vi "CONFOCAL MICROSCOPE.vi"() -> ()   [LabVIEW 2025]
uses:
  <vilib>/Analysis/1siggen.llb/Ramp Pattern by Samples.vi
  <vilib>/DAQmx/write.llb/DAQmx Write (Analog 1D Wfm NChan NSamp).vi
  <vilib>/DAQmx/read.llb/DAQmx Read (Counter 1D U32 1Chan NSamp).vi
  <vilib>/DAQmx/create/channels.llb/DAQmx Create Channel (AO-Voltage-Basic).vi
  <vilib>/DAQmx/configure/timing.llb/DAQmx Timing (Sample Clock).vi
  <vilib>/DAQmx/configure/events/hardwareSignals.llb/DAQmx Export Signal (Most Signals).vi
  <vilib>/DAQmx/miscellaneous.llb/DAQmx Fill In Error Info.vi
  <vilib>/DAQmx/create/channels.llb/DAQmx Create Channel (CI-Count Edges).vi
  <vilib>/Analysis/NI_AALBase.lvlib
panel:
  out "Sanning \nhas\nstarted":bool
  in  "Info Filling":bool
  in  "Length of the material":dbl
  in  "Objective magnification":dbl
  in  "Imaging focal length":dbl
  in  "Scaling factor":dbl
  in  "Pixel per line (X and Y)":dbl
  out "Resolution limit exceeded":bool
  out "transposed array":dbl[][](array[numeric])
  out "Intensity Graph":dbl[][](graph)
  out "Min Voltage (V)":dbl
  out "Max Voltage (V)":dbl
  in  "Dwell time (s)":dbl
  in  "Galvo mirror path":string
  in  "Sample mode":i32(ring)=10178 items=["Finite Samples"=10178, "Continuous Samples"=10123, "Hardware Timed Single Point"=12522]
  out "appended array":dbl[][](array[numeric])
  in  "Counter path":string
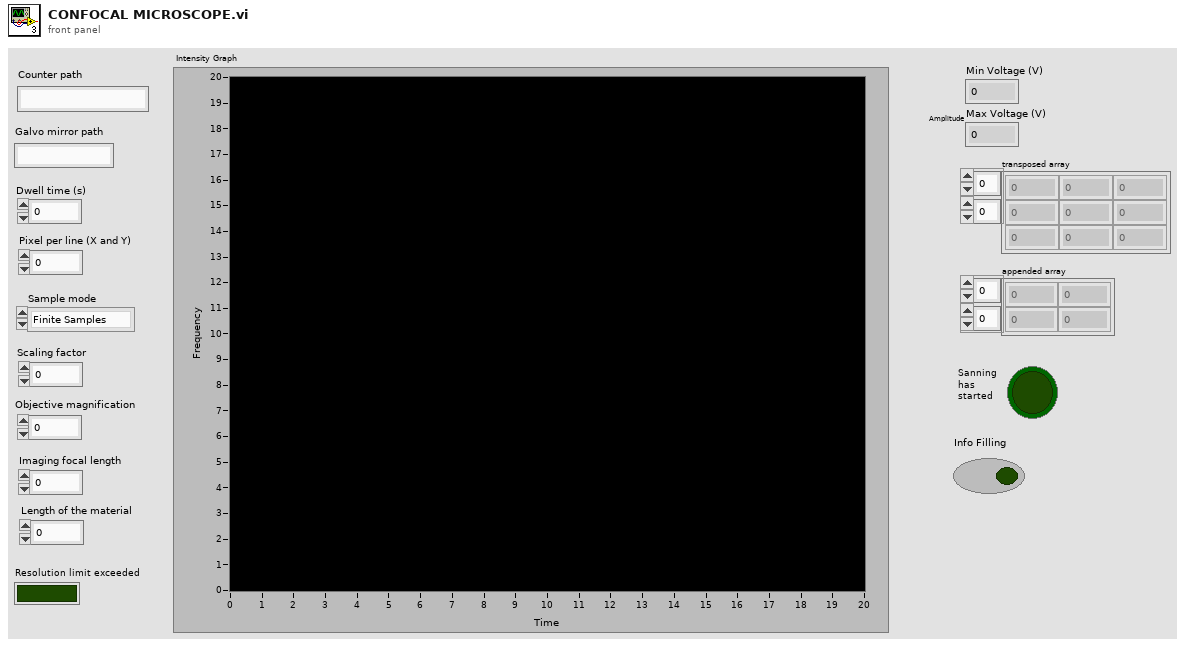
[diagram p1: front panel]
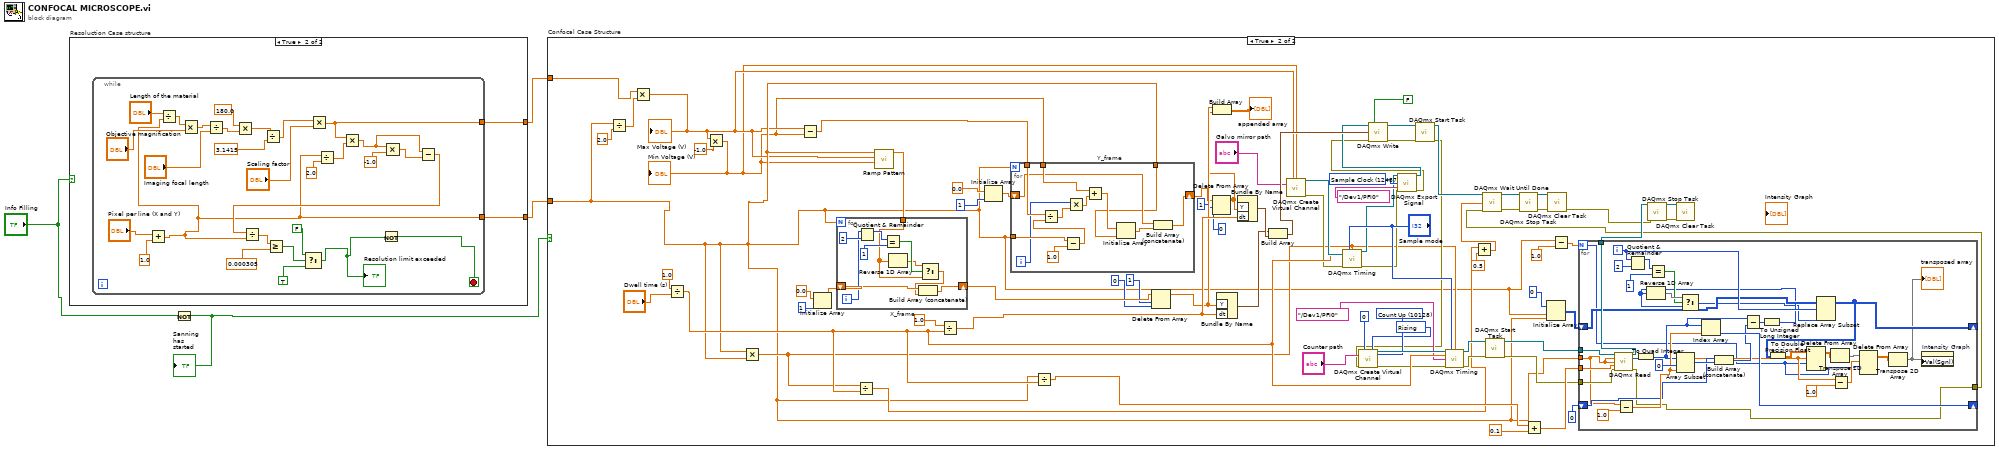
[diagram p0: block diagram]
diagram:
  n1 = case "Resoluction Case structure" shown="True" "Info Filling" {
    tunnel: [_ w5] -> w4
    tunnel: [_ w6] -> w3
    frame False {
    }
    frame True {
      n2 = while {
        tunnel: [w18] -> w6
        tunnel: [w7] -> w5
        stop <- w10 stop-if-true
        n3 = Add(x="Pixel per line (X and Y)", y=1.0) -> (x+y=w7:dbl)
        n4 = Divide(x="Length of the material", y=w7) -> (x/y=w33:dbl)
        n5 = Multiply(x=w33, y="Objective magnification") -> (x*y=w31:dbl)
        n6 = Divide(x=w31, y="Imaging focal length") -> (x/y=w28:dbl)
        n7 = Multiply(x=180.0, y=w28) -> (x*y=w27:dbl)
        n8 = Divide(x=w27, y=3.1415) -> (x/y=w25:dbl)
        n9 = Multiply(x=w25, y="Scaling factor") -> (x*y=w18:dbl)
        n10 = Divide(x=w7, y=2.0) -> (x/y=w17:dbl)
        n11 = Multiply(x=w18, y=w17) -> (x*y=w13:dbl)
        n12 = Multiply(x=w13, y=-1.0) -> (x*y=w14:dbl)
        n13 = Subtract(x=w13, y=w14) -> (x-y=w12:dbl)
        n14 = Divide(x=w12, y=w7) -> (x/y=w23:dbl)
        n15 = Greater Or Equal?(x=w23, y=0.000305) -> (x >= y?=w21:bool)
        n16 = Select(t=FALSE, s=w21, f=TRUE) -> (s? t:f=w11:bool)
        "Resolution limit exceeded" <- w11
        n17 = Not(x=w11) -> (.not. x?=w10:bool)
      }
    }
  }
  n18 = Not(x="Info Filling") -> (.not. x?=w1:bool)
  "Sanning \nhas\nstarted" <- w1
  n19 = case "Confocal Case Structure" shown="True" w1 {
    tunnel: w4 -> [_ w38]
    tunnel: w3 -> [_ w39]
    frame False {
    }
    frame True {
      w79 = 12487 items=["AI Convert Clock"=12484, "10MHz Reference Clock"=12536, "20MHz Timebase Clock"=12486, "Sample Clock"=12487, "Advance Trigger"=12488, "Reference Trigger"=12490, "Start Trigger"=12491, "Advance Complete Event"=12492, "AI Hold Complete Event"=12493, "Counter Output Event"=12494, "Change Detection Event"=12511, "Watchdog Timer Expired Event"=12512] ("signal")
      w84 = 10280 items=["Rising"=10280, "Falling"=10171] ("edge")
      w85 = 10128 items=["Count Up"=10128, "Count Down"=10124, "Externally Controlled"=10326] ("count direction")
      n20 = Divide(x=w38, y=2.0) -> (x/y=w41:dbl)
      n21 = Multiply(x=w39, y=w41) -> (x*y=w36:dbl)
      "Max Voltage (V)" <- w36
      n22 = Divide(x=1.0, y="Dwell time (s)") -> (x/y=w64:dbl)
      n23 = Multiply(x=w36, y=-1.0) -> (x*y=w35:dbl)
      "Min Voltage (V)" <- w35
      n24 = Multiply(x=w38, y=w38) -> (x*y=w45:dbl)
      n25 = Subtract(x=w36, y=w35) -> (x-y=w81:dbl)
      n26 = Initialize Array(0.0 ("element"), 1 ("dimension size")) -> (w92:dbl[])
      n27 = Divide(x=w45, y=w64) -> (x/y=w44:dbl)
      n28 = call-poly <vilib>:"Ramp Pattern.vi"("start"=w35, "end"=w36, "samples"=w38) -> ("Ramp Pattern"=w109:dbl[])  [unwired: 7 in, 1 out]
      n29 = for "X_frame" {
        N: w38 -> [_]
        shift-right: [w169] -> w75
        shift-left: w92 -> [w170]
        tunnel: w109 -> [w163]
        i -> [w164]
        n30 = Quotient & Remainder(x=w164, y=2) -> (x-y*floor(x/y)=w167:i32)  [unwired: 1 out]
        n31 = Equal?(x=w167, y=1) -> (x = y?=w165:bool)
        n32 = Reverse 1D Array(array=w163) -> (reversed array=w162:dbl[])
        n33 = Select(t=w162, s=w165, f=w163) -> (s? t:f=w161:dbl[])
        n34 = Build Array (concatenate)(w170, w161) -> (w169:dbl[])
      }
      n35 = Divide(x=1.0, y=w64) -> (x/y=w94:dbl)
      n36 = Initialize Array(0.0 ("element"), 1 ("dimension size")) -> (w93:dbl[])
      n37 = for "Y_frame" {
        N: w38 -> [_]
        tunnel: w38 -> [w160]
        tunnel: w81 -> [w158]
        tunnel: w35 -> [w153]
        tunnel: w38 -> [w148]
        shift-right: [w149] -> w71
        shift-left: w93 -> [w150]
        i -> [w155]
        n38 = Subtract(x=w160, y=1.0) -> (x-y=w157:dbl)
        n39 = Divide(x=w158, y=w157) -> (x/y=w156:dbl)
        n40 = Multiply(x=w155, y=w156) -> (x*y=w154:dbl)
        n41 = Add(x=w153, y=w154) -> (x+y=w152:dbl)
        n42 = Initialize Array(w152, w148) -> (w151:dbl[])
        n43 = Build Array (concatenate)(w150, w151) -> (w149:dbl[])
      }
      n44 = Divide(x=w38, y=w64) -> (x/y=w60:dbl)
      n45 = Delete From Array "Delete From Array"(array=w75, length=1, index=0) -> (array with subset deleted=w72:dbl[])  [unwired: 1 out]
      n46 = Delete From Array "Delete From Array"(array=w71, length=1, index=0) -> (array with subset deleted=w65:dbl[])  [unwired: 1 out]
      n47 = Build Array(w72, w65) -> (→"appended array":dbl[][])
      n48 = Bundle By Name("Y"=w72, "dt"=w94) -> (w95:waveform(dbl))  [unwired: 1 in]
      n49 = Bundle By Name("Y"=w65, "dt"=w94) -> (w96:waveform(dbl))  [unwired: 1 in]
      n50 = Build Array(w95, w96) -> (w99:waveform(dbl)[])
      n51 = call-poly <vilib>:"DAQmx Create Virtual Channel.vi"("maximum value"=w36, "minimum value"=w35, "physical channels"="Galvo mirror path") -> ("task out"=w98:refnum<k21>, "error out"=w58:errorcluster)  [unwired: 11 in]
      n52 = call-poly <vilib>:"DAQmx Timing.vi"("task/channels in"=w98, "sample mode"="Sample mode", "samples per channel"=w45, "rate"=w64, "error in"=w58) -> ("task out"=w77:refnum<k21>, "error out"=w57:errorcluster)  [unwired: 9 in]
      n53 = call-poly <vilib>:"DAQmx Export Signal.vi"("task/channels in"=w77, "signal"=w79, "output terminal"=tag "/Dev1/PFI0", "error in"=w57) -> ("task out"=w76:refnum<k21>, "error out"=w56:errorcluster)  [unwired: 10 in]
      n54 = call-poly <vilib>:"DAQmx Write.vi"("task/channels in"=w76, "auto start"=FALSE, "data"=w99, "error in"=w56) -> ("task out"=w100:refnum<k21>, "error out"=w55:errorcluster)  [unwired: 9 in, 1 out]
      n55 = call <vilib>:"DAQmx Start Task.vi"("task/channels in"=w100, "error in"=w55) -> ("task out"=w107:refnum<k21>, "error out"=w52:errorcluster)  [unwired: 12 in]
      n56 = call-poly <vilib>:"DAQmx Create Virtual Channel.vi"("initial count"=u32 0, "count direction"=w85, "edge"=w84, "counter"="Counter path", "error in"=w52) -> ("task out"=w102:refnum<k21>, "error out"=w54:errorcluster)  [unwired: 9 in]
      n57 = call-poly <vilib>:"DAQmx Timing.vi"("task/channels in"=w102, "sample mode"="Sample mode", "samples per channel"=w45, "rate"=w64, "source"=tag "/Dev1/PFI0", "error in"=w54) -> ("task out"=w103:refnum<k21>, "error out"=w53:errorcluster)  [unwired: 8 in]
      n58 = Add(x=w44, y=0.5) -> (x+y=w42:dbl)
      n59 = call <vilib>:"DAQmx Start Task.vi"("task/channels in"=w103, "error in"=w53) -> ("task out"=w104:refnum<k21>, "error out"=w47:errorcluster)  [unwired: 12 in]
      n60 = Add(x=w60, y=0.1) -> (x+y=w66:dbl)
      n61 = Initialize Array(u32 0 ("element"), w38, w38) -> (w106:u32[][])
      n62 = Subtract(x=w38, y=1.0) -> (x-y=w62:dbl)
      n63 = for {
        N: w62 -> [w116]
        tunnel: w38 -> [w119]
        tunnel: w66 -> [w147]
        tunnel: w104 -> [w146]
        shift-right: [w127] -> _
        shift-left: w106 -> [w130]
        tunnel: [w141] -> w59
        shift-right: [w136] -> _
        shift-left: u64 0 ("Numeric") -> [w134]
        tunnel: w47 -> [w124]
        tunnel: [w123] -> w46
        i -> [w131]
        n64 = call-poly <vilib>:"DAQmx Read.vi"("task/channels in"=w146, "number of samples per channel"=w119, "timeout"=w147, "error in"=w124) -> ("task out"=w141:refnum<k21>, "data"=w126:u32[], "error out"=w123:errorcluster)  [unwired: 9 in]
        n65 = Subtract(x=w119, y=1.0) -> (x-y=w135:dbl)
        n66 = Quotient & Remainder(x=w131, y=2) -> (x-y*floor(x/y)=w144:i32)  [unwired: 1 out]
        n67 = To Quad Integer(1:w126) -> (0:w125:i64[])
        n68 = Equal?(x=w144, y=1) -> (x = y?=w140:bool)
        n69 = Array Subset "Array Subset"(array=w125, index=0, length=w135) -> (w137:i64[])
        n70 = Index Array "Index Array"(array=w125, index=w135) -> (element=w136:i64)
        n71 = Build Array (concatenate) "Build Array"(w134, w137) -> (w133:u64[])
        n72 = Subtract(x=w125, y=w133) -> (x-y=w132:u64[])
        n73 = To Unsigned Long Integer(number=w132) -> (unsigned 32bit integer=w129:u32[])
        n74 = Reverse 1D Array(array=w129) -> (reversed array=w142:u32[])
        n75 = Select(t=w142, s=w140, f=w129) -> (s? t:f=w128:u32[])
        n76 = Replace Array Subset "Replace Array Subset"(array=w130, new element=w128, index (row)=w131) -> (w127:u32[][])  [unwired: 1 in]
        n77 = To Double Precision Float(number=w127) -> (double precision float=w122:dbl[][])
        n78 = Delete From Array(array=w122, length=w119, index (row)=w116) -> (array with subset deleted=w121:dbl[][])  [unwired: 1 in, 1 out]
        n79 = Transpose 2D Array(2D array=w121) -> (transposed array=w120:dbl[][])
        n80 = Subtract(x=w119, y=1.0) -> (x-y=w117:dbl)
        n81 = Delete From Array(array=w120, length=w117, index (row)=w116) -> (array with subset deleted=w115:dbl[][])  [unwired: 1 in, 1 out]
        n82 = Transpose 2D Array(2D array=w115) -> (transposed array=w114:dbl[][])
        "transposed array" <- w114
        n83 = property on="Intensity Graph" class="IntGraph (strict)"("Val(Sgnl)"=w114) -> ()  [unwired: 2 in, 2 out]
      }
      n84 = call <vilib>:"DAQmx Wait Until Done.vi"("task/channels in"=w107, "timeout (sec)"=w42, "error in"=w46) -> ("task out"=w108:refnum<k21>, "error out"=w51:errorcluster)  [unwired: 11 in]
      n85 = call <vilib>:"DAQmx Stop Task.vi"("task/channels in"=w108, "error in"=w51) -> ("task out"=w101:refnum<k21>, "error out"=w50:errorcluster)  [unwired: 12 in]
      n86 = call <vilib>:"DAQmx Clear Task.vi"("task in"=w101, "error in"=w50) -> ("error out"=w49:errorcluster)  [unwired: 13 in]
      n87 = call <vilib>:"DAQmx Stop Task.vi"("task/channels in"=w59, "error in"=w49) -> ("task out"=w110:refnum<k21>, "error out"=w48:errorcluster)  [unwired: 12 in]
      n88 = call <vilib>:"DAQmx Clear Task.vi"("task in"=w110, "error in"=w48) -> ()  [unwired: 13 in, 1 out]
    }
  }
